vi "StartVideo fullscreen.vi"(0 "VLC Variables In":T1, 1 "PictureBox":refnum<k24>(container), 9 "Media Source":string="dshow://", 11 "error in (no error)":errorcluster) -> (4 "VLC Variables Out":T1, 15 "error out":errorcluster)   [LabVIEW 2012]
doc: "Set up all option to start streaming video from the webcam"
uses:
  Controls-Webcam/VLC Var.ctl
  System.Windows.Forms
panel:
  in  "Script":string
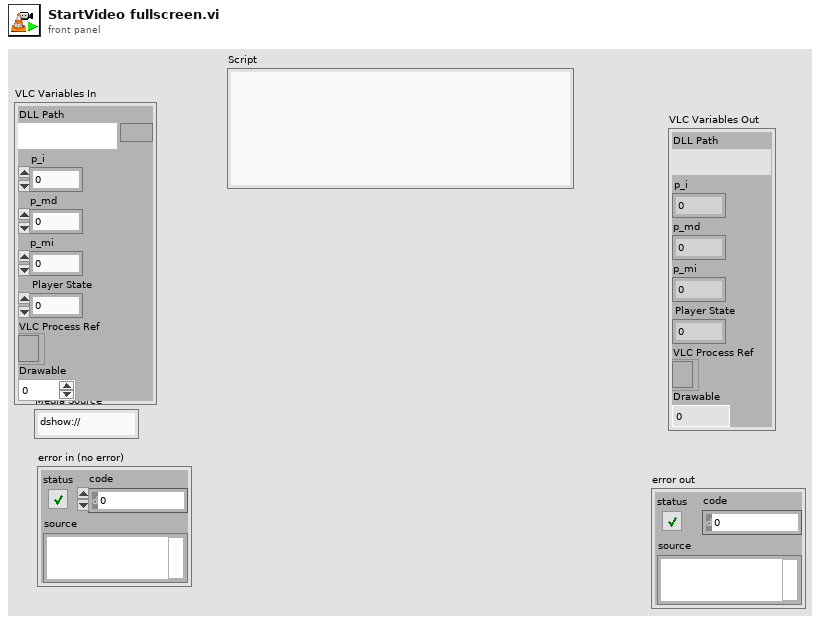
[diagram p1: front panel]
types:
  T1 = typedef "VLC Var.ctl" = cluster{"DLL Path":path, "p_i":i32, "p_md":i32, "p_mi":i32, "Player State":i32, "VLC Process Ref":refnum<k24>, "Drawable":i32}
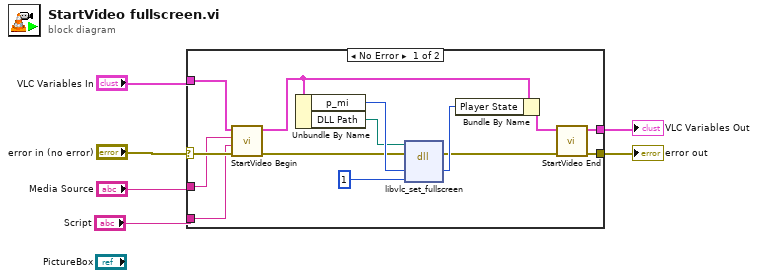
[diagram p0: block diagram]
diagram:
  n1 = case shown="No Error" "error in (no error)" {
    selector: "error in (no error)" -> [w10 w22]
    tunnel: [w18 w21] -> w6
    tunnel: [w17 w22] -> w5
    tunnel: "VLC Variables In" -> [w9 w21]
    tunnel: "Media Source" -> [w8 _]
    tunnel: "Script" -> [w7 _]
    frame No Error {
      n2 = call "StartVideo Begin.vi"("error in (no error)"=w10, "Script"=w7, "Media Source"=w8, "VLC Variables In in"=w9) -> ("error out"=w11:errorcluster, "VLC Variables In out"=w12:T1)  [unwired: 6 in]
      n3 = Unbundle By Name(w12) -> ("p_mi"=w19:i32, "DLL Path"=w13:path)
      n4 = dll-call lib="C:/Program Files (x86)/VideoLAN/VLC/libvlc.dll" fn="libvlc_set_fullscreen"(path in=w13, error in=w11, "p_mi"=w19, "fullscreen"=1) -> (error out=w14:errorcluster, "p_mi"=w16:i32)  [unwired: 3 in, 1 out]
      n5 = Bundle By Name(cluster=w12, "Player State"=w16) -> (w15:T1)
      n6 = call "StartVideo End.vi"("error in (no error)"=w14, "VLC Variables In in"=w15) -> ("error out"=w17:errorcluster, "VLC Variables In out"=w18:T1)  [unwired: 8 in]
    }
    frame Error {
    }
  }
  "error out" <- w5
  "VLC Variables Out" <- w6
